vi "VI.open_fp_lua.vi"(5 "LuaVIEW reference":T1) -> (15 "error out":errorcluster)   [LabVIEW 2012]
doc: "Opens the front panel of a VI. This method maps to the LabVIEW open fp VI method. When the front panel is already open it will be brought to the front.\nParameters:\nobj:self, object of the VI.\n[bool:activate], determines whether the front panel should be activated on opening. Defaults to true when not specified.\nErrors:\nNot a VI object.\nDead VI object.\nCould not open front panel."
uses:
  typedefs/t_LuaVIEW Reference.ctl
  subvis/private/LuaVIEW Pull (object).vi
  subvis/private/LuaVIEW Pull (boolean).vi
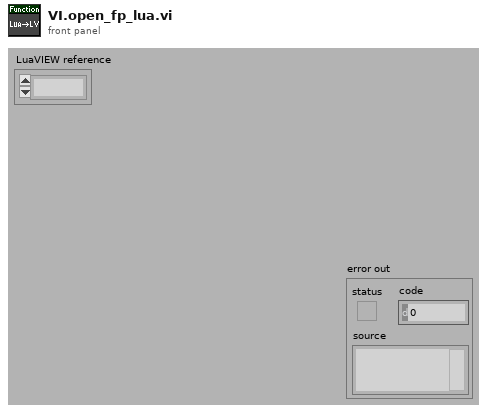
[diagram p1: front panel]
types:
  T1 = typedef "t_LuaVIEW Reference.ctl" = refnum<k1>
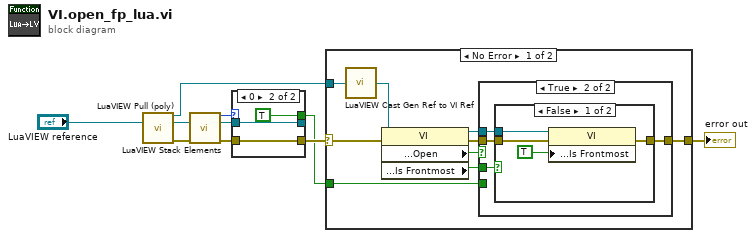
[diagram p0: block diagram]
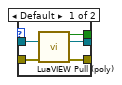
[diagram p2: hidden frame]
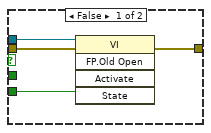
[diagram p3: hidden frame]
diagram:
  n1 = call-poly "LuaVIEW Pull (poly).vi"("LuaVIEW reference in"="LuaVIEW reference") -> ("object refnum"=w1:refnum<vi>, "LuaVIEW reference out"=w4:T1, "error out"=w5:errorcluster)  [unwired: 11 in, 1 out]
  n2 = call "LuaVIEW Stack Elements.vi"("LuaVIEW reference in"=w4, "error in (no error)"=w5) -> ("elements"=w8:i32, "LuaVIEW reference out"=w6:T1, "error out"=w7:errorcluster)  [unwired: 11 in]
  n3 = case shown="0" w8 {
    tunnel: w7 -> [w15 w17]
    tunnel: w6 -> [w14 w18]
    tunnel: [w13 w18] -> _
    tunnel: [w12 TRUE ("boolean")] -> w2
    tunnel: [w11 w17] -> w3
    frame Default {
      n4 = call-poly "LuaVIEW Pull (poly).vi"("LuaVIEW reference in"=w14, "error in (no error)"=w15) -> ("boolean"=w12:bool, "LuaVIEW reference out"=w13:T1, "error out"=w11:errorcluster)  [unwired: 11 in]
    }
    frame 0 {
    }
  }
  n5 = case shown="No Error" w3 {
    selector: w3 -> [w25 w41]
    tunnel: [w27 w41] -> w9
    tunnel: w2 -> [w23 _]
    tunnel: w1 -> [w26 _]
    frame No Error {
      n6 = call "LuaVIEW Cast Gen Ref to VI Ref.vi"("refnum in"=w26) -> ("refnum out"=w24:refnum<vi>)  [unwired: 14 in]
      n7 = property class="VI"(reference=w24, error in=w25) -> (reference out=w22:refnum<vi>, error out=w21:errorcluster, "Front Panel Window:Open"=w20:bool, "Front Panel Window:Is Frontmost"=w19:bool)
      n8 = case shown="True" w20 {
        tunnel: [w31 w35] -> w27
        tunnel: w23 -> [w30 _]
        tunnel: w22 -> [w29 w33]
        tunnel: w21 -> [w28 w32]
        tunnel: w19 -> [_ w34]
        frame False {
          n9 = invoke class="VI" method="FP.Old Open"(reference=w29, error in=w28, "Activate"=w30) -> (error out=w31:errorcluster)  [unwired: 2 in, 4 out]
        }
        frame True {
          n10 = case shown="False" w34 {
            tunnel: [w39 w40] -> w35
            tunnel: w33 -> [w38 _]
            tunnel: w32 -> [w37 w40]
            frame False {
              n11 = property class="VI"(reference=w38, error in=w37, "Front Panel Window:Is Frontmost"=TRUE) -> (error out=w39:errorcluster)  [unwired: 1 out]
            }
            frame True {
            }
          }
        }
      }
    }
    frame Error {
    }
  }
  "error out" <- w9
